vi "SystemParams.vi"(0 "System Up Time In":u32, 1 "Unit Add":u32, 3 "RingCancelDelay":u32 format="%.0x", 4 "Vin High Th":dbl, 5 "Op Amp Gain in":u32, 7 "Vin Low Th":dbl, 8 "aDATA":u8[](array[numeric]), 9 "R Sense [Ohms] in":u32, 10 "Temp High Th":dbl, 11 "String":string, 12 "Temp Low Th":dbl) -> (16 "Temp Low Th out":dbl, 17 "Vin Low Th out":dbl, 18 "Temp High Th out":dbl, 19 "String out":string, 20 "System Up Time  Out":u32, 21 "Unit Add Out":u32, 23 "RingCancelDelay out":u32 format="%.0x", 24 "Vin High Th out":dbl, 25 "R Sense [Ohms] out":u32, 27 "Op Amp Gain out":u32)   [LabVIEW 2017]
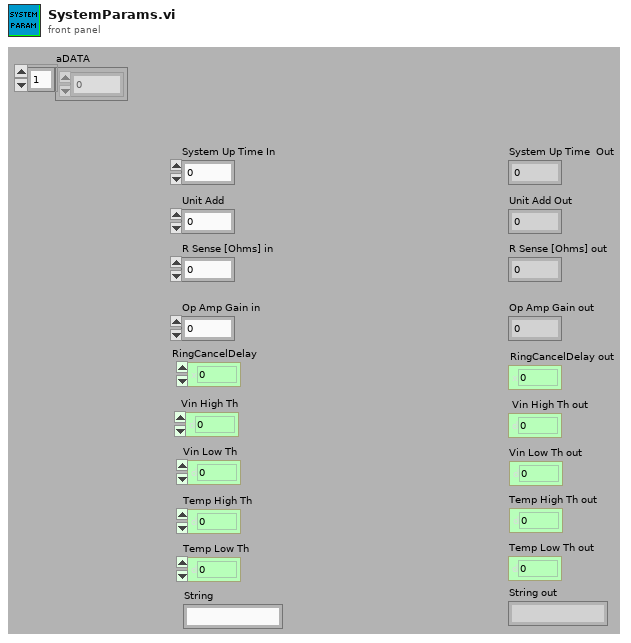
[diagram p1: front panel]
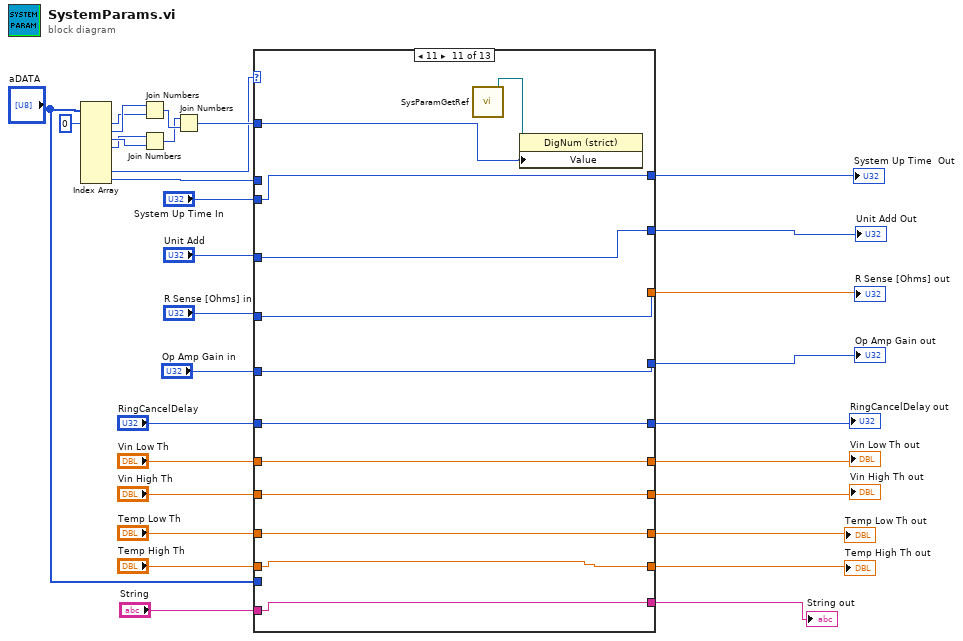
[diagram p0: block diagram]
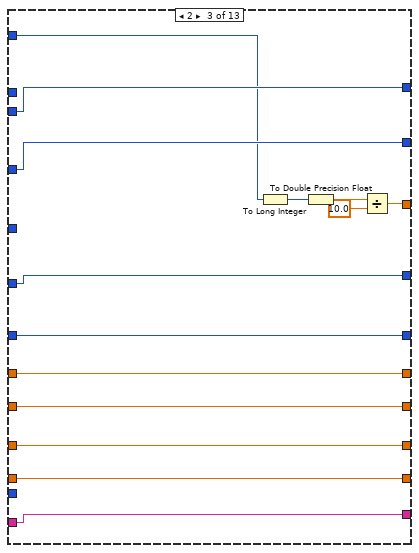
[diagram p4: hidden frame]
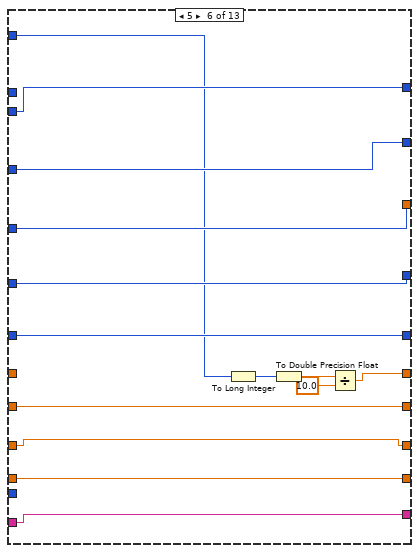
[diagram p7: hidden frame]
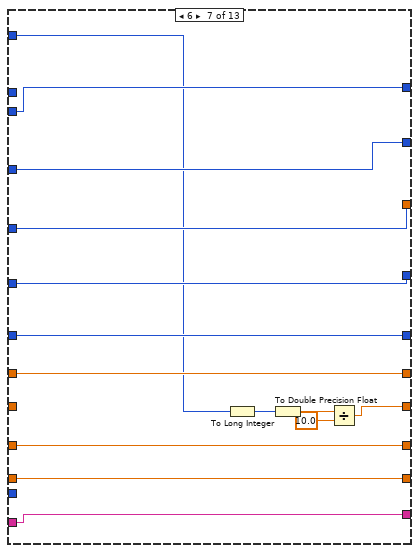
[diagram p8: hidden frame]
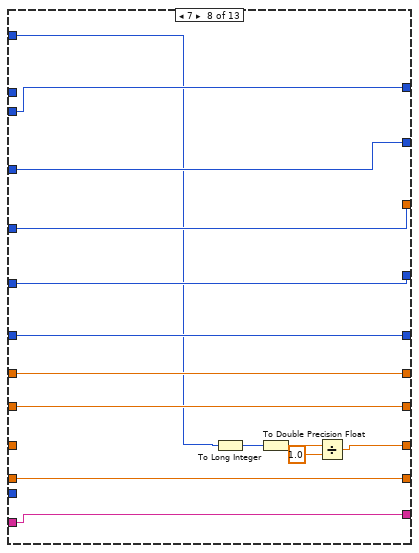
[diagram p9: hidden frame]
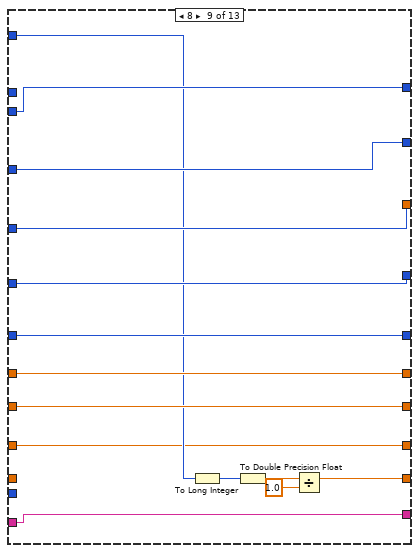
[diagram p10: hidden frame]
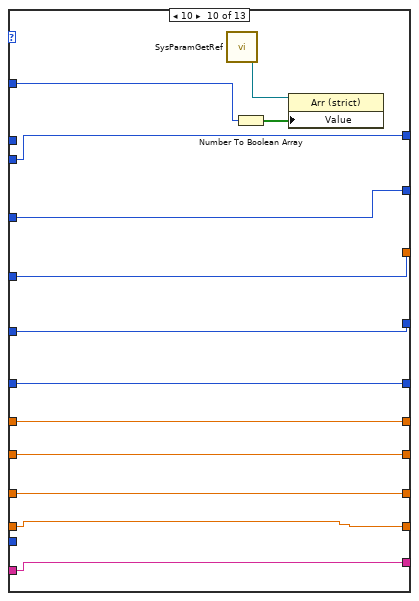
[diagram p11: hidden frame]
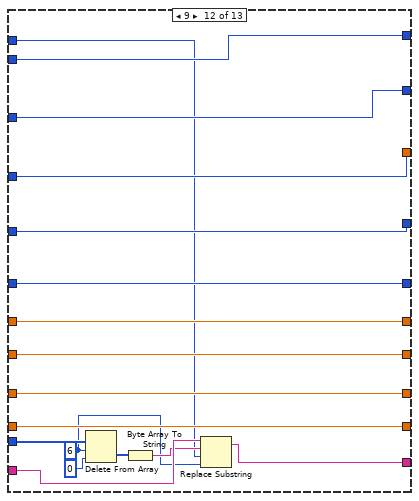
[diagram p12: hidden frame]
diagram:
  n1 = Index Array(array="aDATA", index #1=0 ("index")) -> (element #1=w26:u8, element #2=w27:u8, element #3=w29:u8, element #4=w28:u8, element #7=w2:u8, element #8=w1:u8)  [unwired: 7 in, 2 out]
  n2 = Join Numbers(hi=w27, lo=w26) -> ((hi.lo)=w31:u16)
  n3 = Join Numbers(hi=w28, lo=w29) -> ((hi.lo)=w30:u16)
  n4 = Join Numbers(hi=w30, lo=w31) -> ((hi.lo)=w24:u32)
  n5 = case shown="11" w2 {
    tunnel: w24 -> [w39 w48 w53 w72 w79 w87 w101 w115 w133 w143 w155 _ _]
    tunnel: [w39 w51 w65 w75 w85 w99 w113 w127 w141 w154 w166 w183 w193] -> w22
    tunnel: "System Up Time In" -> [_ w51 w65 w75 w85 w99 w113 w127 w141 w154 w166 w183 w193]
    tunnel: "Unit Add" -> [w38 _ w64 w74 w84 w98 w112 w126 w140 w153 w165 w182 w192]
    tunnel: [w38 w48 w64 w74 w84 w98 w112 w126 w140 w153 w165 w182 w192] -> w21
    tunnel: [w41 w50 w52 w73 w83 w97 w111 w125 w139 w152 w164 w181 w191] -> w20
    tunnel: "R Sense [Ohms] in" -> [w41 w50 _ w73 w83 w97 w111 w125 w139 w152 w164 w181 w191]
    tunnel: "Op Amp Gain in" -> [w40 w49 w63 _ w82 w96 w110 w124 w138 w151 w163 w180 w190]
    tunnel: [w40 w49 w63 w72 w82 w96 w110 w124 w138 w151 w163 w180 w190] -> w18
    tunnel: "RingCancelDelay" -> [w37 w47 w62 w71 _ w94 w109 w123 w137 w150 w162 w179 w189]
    tunnel: [w37 w47 w62 w71 w79 w94 w109 w123 w137 w150 w162 w179 w189] -> w14
    tunnel: "Vin Low Th" -> [w36 w46 w61 w70 w81 _ w108 w122 w136 w149 w161 w178 w188]
    tunnel: [w36 w46 w61 w70 w81 w86 w108 w122 w136 w149 w161 w178 w188] -> w12
    tunnel: "Vin High Th" -> [w35 w45 w60 w69 w80 w95 _ w119 w134 w147 w159 w177 w187]
    tunnel: [w35 w45 w60 w69 w80 w95 w100 w119 w134 w147 w159 w177 w187] -> w10
    tunnel: "Temp Low Th" -> [w34 w44 w59 w68 w78 w93 w107 _ w132 w146 w158 w176 w185]
    tunnel: "Temp High Th" -> [w33 w43 w58 w67 w77 w92 w106 w121 _ w145 w157 w175 w184]
    tunnel: [w32 w42 w57 w66 w76 w91 w105 w120 w135 w148 w160 w168 w186] -> w4
    tunnel: "String" -> [w32 w42 w57 w66 w76 w91 w105 w120 w135 w148 w160 w172 w186]
    tunnel: [w34 w44 w59 w68 w78 w93 w107 w114 w132 w146 w158 w176 w185] -> w6
    tunnel: [w33 w43 w58 w67 w77 w92 w106 w121 w130 w145 w157 w175 w184] -> w5
    tunnel: "aDATA" -> [_ _ _ _ _ _ _ _ _ _ _ w174 _]
    tunnel: w1 -> [_ _ _ _ _ _ _ _ _ _ _ w167 _]
    frame 0 {
    }
    frame 1 {
    }
    frame 2 {
      n6 = To Long Integer(number=w53) -> (32bit integer=w56:i32)
      n7 = To Double Precision Float(number=w56) -> (double precision float=w55:dbl)
      n8 = Divide(x=w55, y=10.0) -> (x/y=w52:dbl)
    }
    frame 3 {
    }
    frame 4 {
    }
    frame 5 {
      n9 = To Long Integer(number=w87) -> (32bit integer=w90:i32)
      n10 = To Double Precision Float(number=w90) -> (double precision float=w89:dbl)
      n11 = Divide(x=w89, y=10.0) -> (x/y=w86:dbl)
    }
    frame 6 {
      n12 = To Long Integer(number=w101) -> (32bit integer=w104:i32)
      n13 = To Double Precision Float(number=w104) -> (double precision float=w103:dbl)
      n14 = Divide(x=w103, y=10.0) -> (x/y=w100:dbl)
    }
    frame 7 {
      n15 = To Long Integer(number=w115) -> (32bit integer=w118:i32)
      n16 = To Double Precision Float(number=w118) -> (double precision float=w117:dbl)
      n17 = Divide(x=w117, y=1.0) -> (x/y=w114:dbl)
    }
    frame 8 {
      n18 = To Long Integer(number=w133) -> (32bit integer=w131:i32)
      n19 = To Double Precision Float(number=w131) -> (double precision float=w129:dbl)
      n20 = Divide(x=w129, y=1.0) -> (x/y=w130:dbl)
    }
    frame 10 {
      n21 = call "SysParamGetRef.vi"() -> ("Sys Tech.Data S out"=w144:refnum<vi>)  [unwired: 16 in, 11 out]
      n22 = Number To Boolean Array(number=w143) -> (Boolean array=w142:bool[])
      n23 = property class="Arr (strict)"(reference=w144, "Value"=w142) -> ()  [unwired: 1 in, 2 out]
    }
    frame 11 {
      n24 = call "SysParamGetRef.vi"() -> ("System Total Time out"=w156:refnum<vi>)  [unwired: 16 in, 11 out]
      n25 = property class="DigNum (strict)"(reference=w156, "Value"=w155) -> ()  [unwired: 1 in, 2 out]
    }
    frame 9 {
      w169 = 6 ("length")
      n26 = Delete From Array(array=w174, length=w169, index=0) -> (deleted portion=w171:u8[])  [unwired: 1 out]
      n27 = Byte Array To String(unsigned byte array=w171) -> (string=w170:string)
      n28 = Replace Substring(2:w169, 3:w167, 4:w170, 5:w172) -> (1:w168:string)  [unwired: 1 out]
    }
    frame 100, Default {
    }
  }
  "System Up Time  Out" <- w22
  "Unit Add Out" <- w21
  "R Sense [Ohms] out" <- w20
  "Op Amp Gain out" <- w18
  "RingCancelDelay out" <- w14
  "Vin Low Th out" <- w12
  "Vin High Th out" <- w10
  "Temp Low Th out" <- w6
  "Temp High Th out" <- w5
  "String out" <- w4
